vi "Excit_Get_Wfm_Name_Binary.vi"(7 "Excit Number":i32, 8 "error in":errorcluster, 9 "Excit Waveforms File Filter":string, 10 "Excit Waveforms Path":path, 11 "Variant":variant) -> (0 "error out":errorcluster caption="sortie d'erreur", 2 "Variant Output":variant, 3 "Waveform Name":string)   [LabVIEW 2018]
doc: "From a start and end value, generates an adiabatic waveform signal of 2000 values (double).\nWrites this waveform into a binary file, in a big-endian format.\nDisplays the written data and the FFT of the signal.\nDefault Path for the generated file is D:\\PIRENEA\\EXCIT_WFMS\n\nAvailable Waveforms : Sinus, Swift, Chirp, Ramp (Up or Down), DoubleRamp (Up-Down or Down-Up)"
uses:
  controls/EXCIT_Waveform_Inputs.ctl
  controls/EXCIT_Form_Selector.ctl
panel:
  in  "EXCIT Waveforms Inputs":T1={"Excit Form"=enum."Swift", "Swift Factor"=0.5, "Chirp Apodisation"=3.5, "Duration"=800.0, "Intensity"=100.0, "Start Frequency"=250.0, "End Frequency"=1000.0, "Intensity 2"=100.0, "Start Frequency 2"=250.0, "End Frequency 2"=350.0, "Sampling Frequency"=10.0} {"End Frequency 2" min=1.0 max=10000.0; "Start Frequency 2" min=1.0 max=10000.0; "Intensity 2" min=1.0 max=100.0; "Chirp Apodisation" min=1.0 max=5.0 step=0.1; "Swift Factor" min=0.1 max=3.0 step=0.1; "Sampling Frequency" min=1.0 max=100.0 step=1.0; "Duration" min=1.0 max=1000000.0 step=1.0; "End Frequency" min=1.0 max=10000.0; "Start Frequency" min=1.0 max=10000.0 step=0.1 format="%#.6g"; "Intensity" min=1.0 max=100.0}
  in  "OK":bool
  out "Excitation FFT":cluster{dbl[], "Power Spectrum (V^2 rms)":dbl[]}(graph)
  out "Excitation Signal":T3(graph)
  out "FIFO used":i32
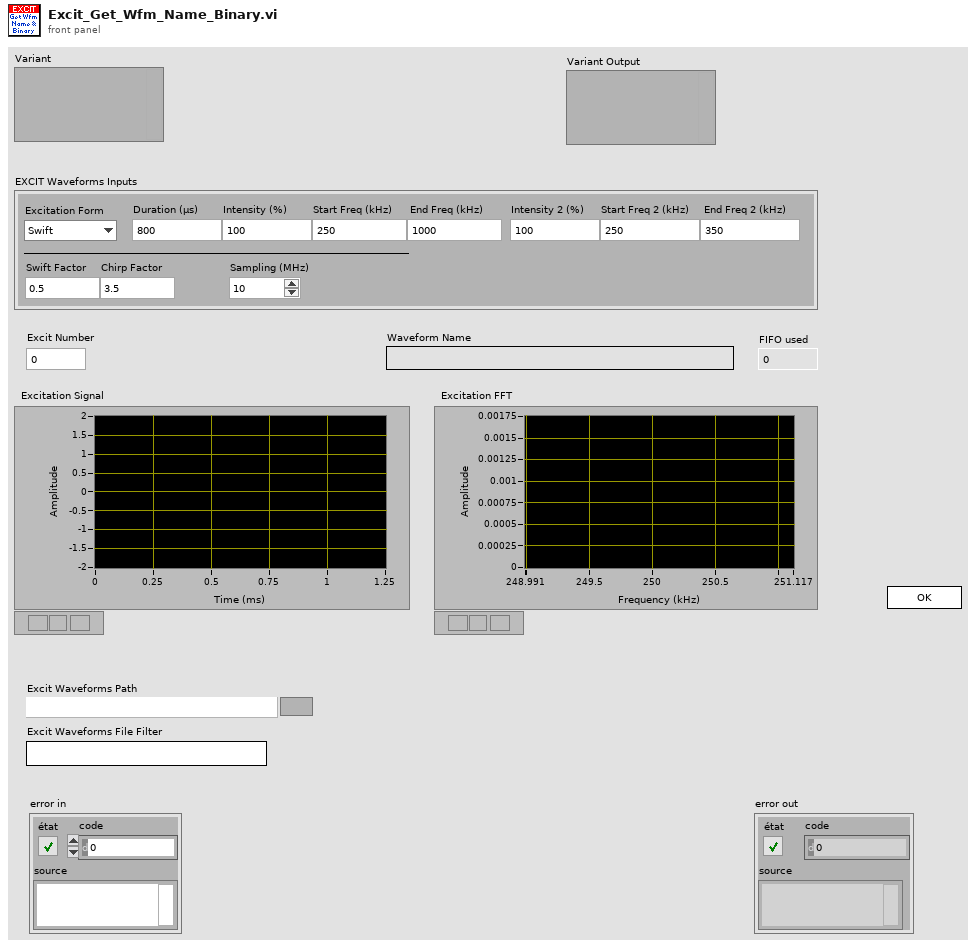
[diagram p1: front panel]
types:
  T1 = typedef "EXCIT_Waveform_Inputs.ctl" = cluster{"Excit Form":T2, "Swift Factor":dbl, "Chirp Apodisation":dbl, "Duration":dbl, "Intensity":dbl, "Start Frequency":dbl, "End Frequency":dbl, "Intensity 2":dbl, "Start Frequency 2":dbl, "End Frequency 2":dbl, "Sampling Frequency":dbl}
  T2 = typedef "EXCIT_Form_Selector.ctl" = enum16{"Swift", "TwoSwift", "Chirp", "Sinus", "Ramp"}
  T3 = cluster{"X Time":dbl[], "Signal Excitation":dbl[]}
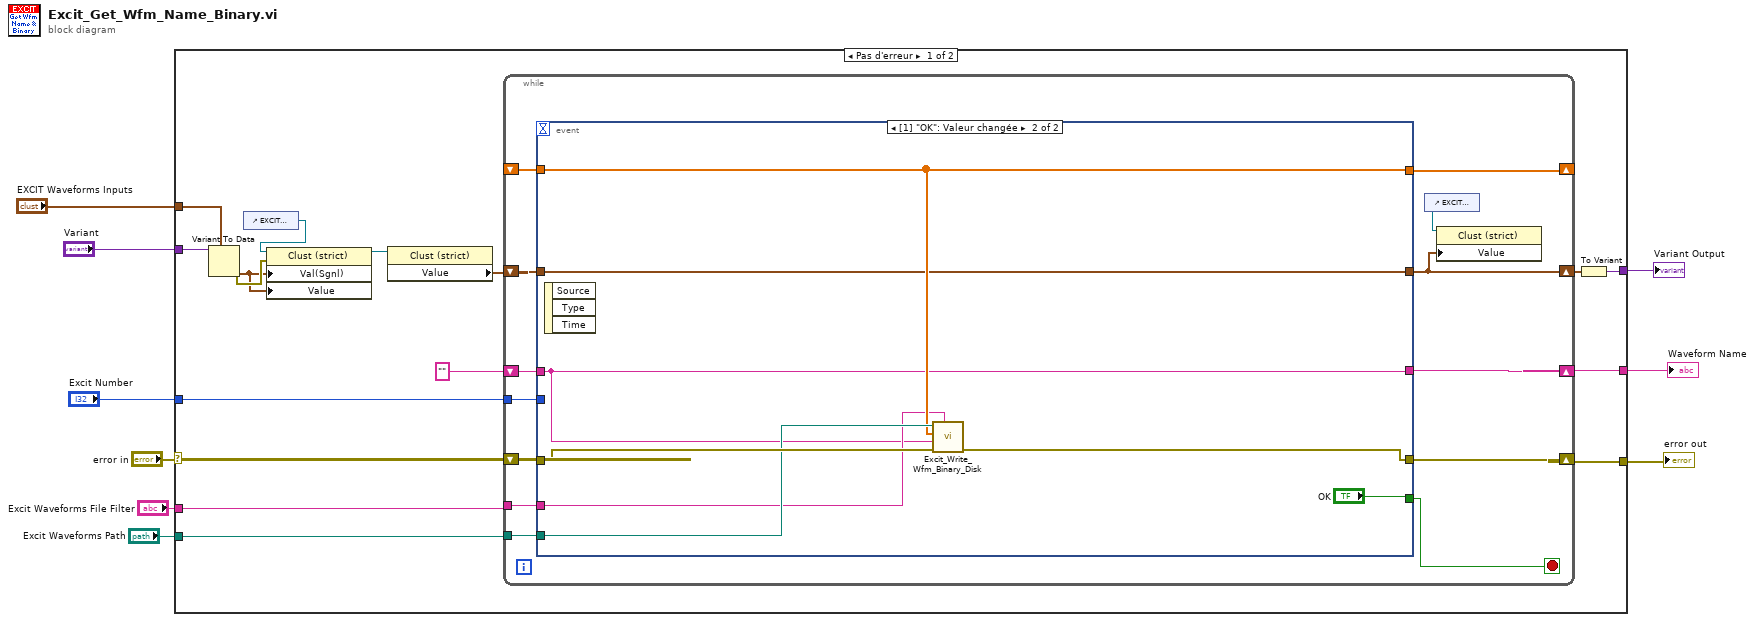
[diagram p0: block diagram]
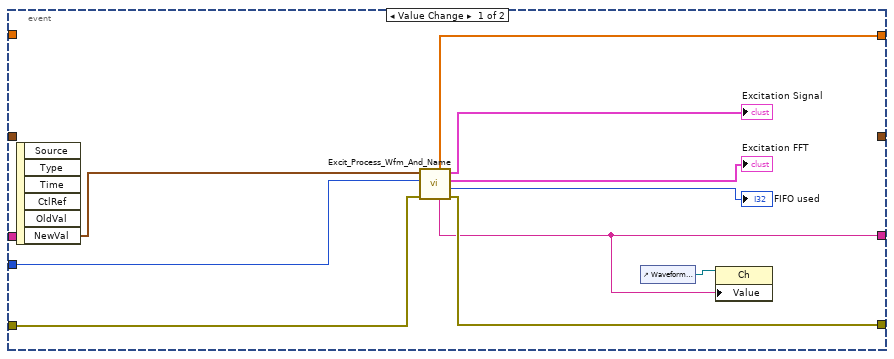
[diagram p2: hidden frame]
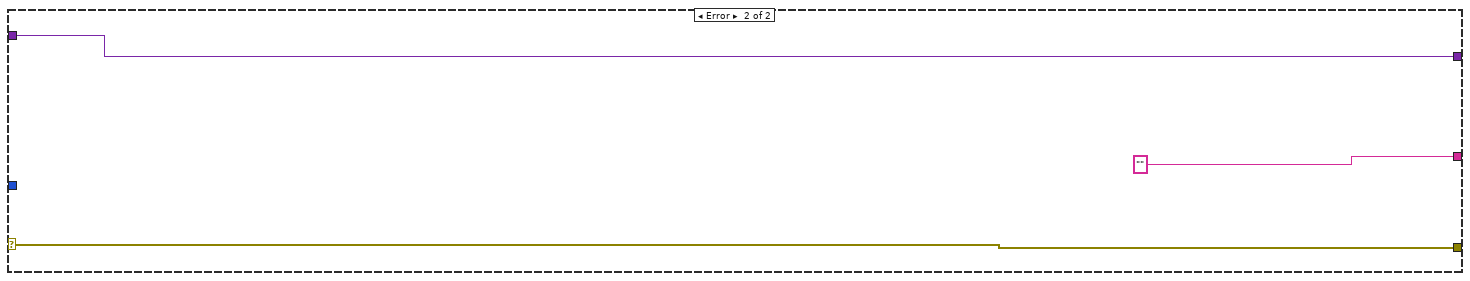
[diagram p3: hidden frame]
diagram:
  n1 = case shown="Pas d'erreur" "error in" {
    selector: "error in" -> [w20 w59]
    tunnel: [w25 w59] -> w9
    tunnel: "Excit Waveforms Path" -> [w24 _]
    tunnel: [w23 ""] -> w1
    tunnel: "Excit Waveforms File Filter" -> [w22 _]
    tunnel: [w16 w57] -> w3
    tunnel: "Excit Number" -> [w19 _]
    tunnel: "Variant" -> [w18 w57]
    tunnel: "EXCIT Waveforms Inputs" -> [w11 _]
    frame No Error {
      n2 = Variant To Data(type=w11, Variant=w18) -> (data=w10:T1, error out=w15:errorcluster)  [unwired: 1 in]
      n3 = control-ref of="EXCIT Waveforms Inputs"() -> (w12:refnum<vi>)
      n4 = property class="Clust (strict)"(reference=w12, error in=w15, "Val(Sgnl)"=w10, "Value"=w10) -> (reference out=w14:refnum<vi>)  [unwired: 1 out]
      n5 = property class="Clust (strict)"(reference=w14) -> ("Value"=w13:T1)  [unwired: 1 in, 2 out]
      n6 = while {
        tunnel: w24 -> [w32]
        shift-right: [w31] -> w25
        shift-left: w20 -> [w38]
        shift-right: [w36] -> _
        shift-left: _ -> [w34]
        shift-right: [w35] -> w23
        shift-left: "" -> [w33]
        tunnel: w22 -> [w30]
        shift-right: [w26] -> w17
        shift-left: w13 -> [w28]
        tunnel: w19 -> [w29]
        stop <- w37 stop-if-true
        n7 = event shown="[1] \"OK\": Valeur changée" {
          selector: _ -> [_ _]
          dyn-events: _ -> [_ _]
          timeout: _ -> [_ _]
          tunnel: [w46 w53] -> w31
          tunnel: w38 -> [w48 w55]
          tunnel: [_ "OK"] -> w37
          tunnel: [w47 w52] -> w36
          tunnel: [w39 w49] -> w35
          tunnel: w34 -> [_ w52]
          tunnel: w33 -> [_ w49]
          tunnel: w32 -> [_ w54]
          tunnel: w30 -> [_ w51]
          tunnel: w29 -> [w41 _]
          tunnel: [_ w50] -> w26
          tunnel: w28 -> [_ w50]
          event Value Change {
            n8 = event-data() -> ("NewVal"=w42:T1)  [unwired: 1 in, 5 out]
            n9 = call "Excit_Process_Wfm_And_Name.vi"("error in (no error)"=w48, "Excit Number"=w41, "EXCIT Waveform Inputs"=w42) -> ("error out"=w46:errorcluster, "FIFO used"=→"FIFO used":i32, "Excitation FFT"=→"Excitation FFT":cluster{dbl[], "Power Spectrum (V^2 rms)":dbl[]}, "Excitation Signal"=→"Excitation Signal":T3, "Waveform Name"=w39:string, "Signal Excitation"=w47:dbl[])  [unwired: 3 in]
            n10 = control-ref of="Waveform Name"() -> (w40:refnum<vi>)
            n11 = property class="Ch"(reference=w40, "Value"=w39) -> ()  [unwired: 1 in, 2 out]
          }
          event "OK": Value Change {
            n12 = event-data() -> ()  [unwired: 1 in, 3 out]
            n13 = call "Excit_Write_Wfm_Binary_Disk.vi"("Excit Waveforms File Filter"=w51, "error in (no error)"=w55, "Waveform Name"=w49, "Signal Excitation"=w52, "Excit Waveforms Path"=w54) -> ("error out"=w53:errorcluster)  [unwired: 6 in]
          }
        }
        n14 = control-ref of="EXCIT Waveforms Inputs"() -> (w27:refnum<vi>)
        n15 = property class="Clust (strict)"(reference=w27, "Value"=w26) -> ()  [unwired: 1 in, 2 out]
      }
      n16 = To Variant(anything=w17) -> (Variant=w16:variant)
    }
    frame Error {
    }
  }
  "error out" <- w9
  "Variant Output" <- w3
  "Waveform Name" <- w1
